vi "MessageBase.setFields.vi"(8 "error in (no error)":errorcluster, 10 "Cluster (dup)":variant, 11 "MessageBase in":refnum<class "MessageBase.lvclass">) -> (0 "error out":errorcluster, 3 "MessageBase out":refnum<class "MessageBase.lvclass">)   [LabVIEW 2022 SP3, in "MessageBase.lvclass"]
uses:
  MessageBase.lvclass
  FieldValue.ctl
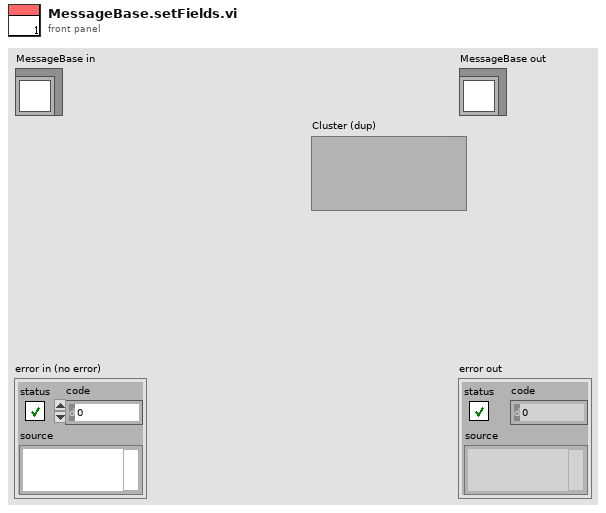
[diagram p1: front panel]
types:
  T1 = typedef "FieldValue.ctl" = variant
  T2 = typedef "FieldSpec.ctl" = cluster{"Name":string, "Offset":i32, "Length":i32, "FieldType":enum16{"Alphanumeric", "Binary", "BinaryLongPrice", "BinaryShortPrice", "BitField", "PrintableAscii", "Value"}, "FieldValue":variant}
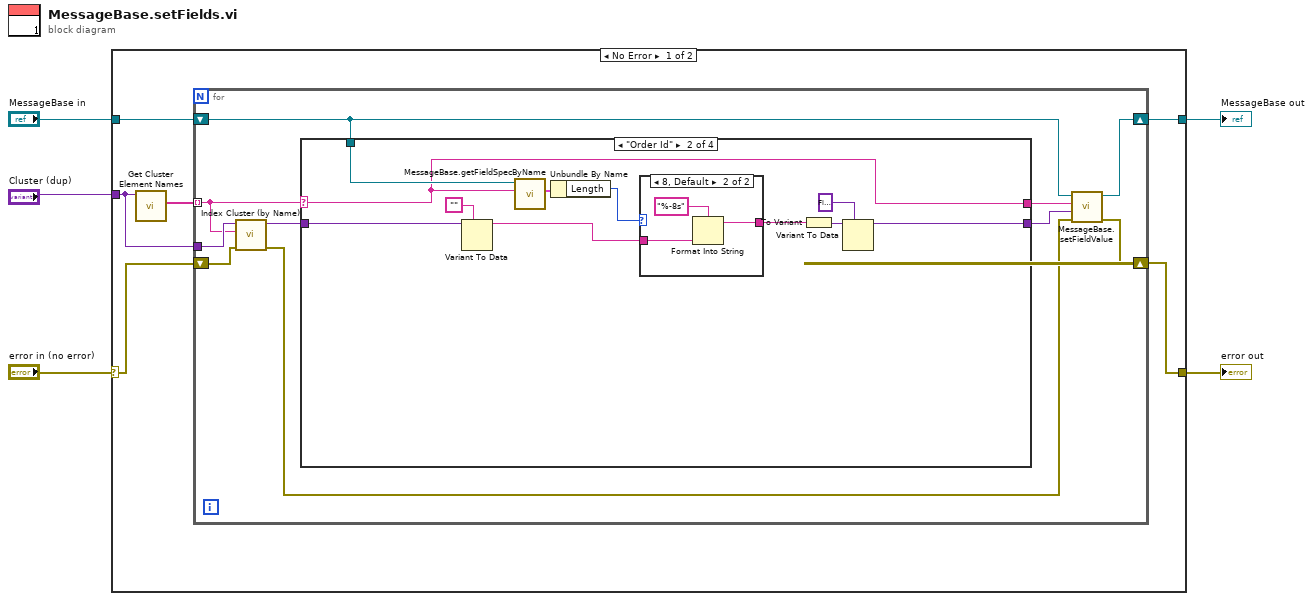
[diagram p0: block diagram]
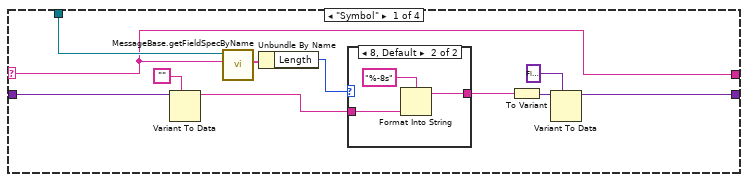
[diagram p2: hidden frame]
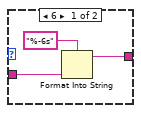
[diagram p3: hidden frame]
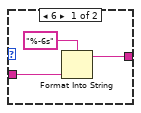
[diagram p4: hidden frame]
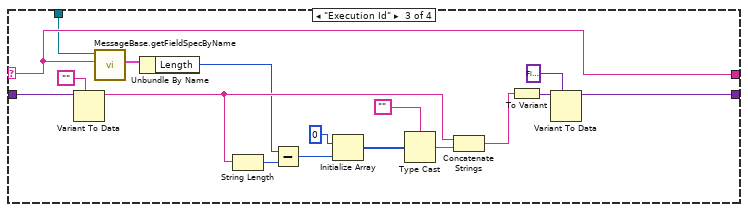
[diagram p5: hidden frame]
diagram:
  n1 = case shown="No Error" "error in (no error)" {
    selector: "error in (no error)" -> [w9 w76]
    tunnel: [w8 w76] -> w4
    tunnel: [w6 w75] -> w2
    tunnel: "MessageBase in" -> [w7 w75]
    tunnel: "Cluster (dup)" -> [w10 _]
    frame No Error {
      n2 = call <vilib>:"Get Cluster Element Names.vi"("Cluster"=w10) -> ("Names"=w11:string[])  [unwired: 8 in, 2 out]
      n3 = for {
        tunnel: w11 -> [w17] mode=indexing
        tunnel: w10 -> [w21]
        shift-right: [w20] -> w6
        shift-left: w7 -> [w12]
        shift-right: [w19] -> w8
        shift-left: w9 -> [w18]
        n4 = call <vilib>:"Index Cluster (by Name).vi"("error in (no error)"=w18, "Element Name"=w17, "Cluster"=w21) -> ("error out"=w13:errorcluster, "Element"=w14:variant)  [unwired: 5 in, 2 out]
        n5 = case shown="\"Order Id\"" w17 {
          selector: w17 -> [w24 w41 w68 w74]
          tunnel: [w24 w41 w68 w74] -> w16
          tunnel: [w30 w47 w70 w73] -> w15
          tunnel: w14 -> [w28 w45 w69 w73]
          tunnel: w12 -> [w25 w42 w56 _]
          frame "Symbol" {
            n6 = Variant To Data(type="", Variant=w28) -> (data=w26:string)  [unwired: 1 in, 1 out]
            n7 = call-dynamic "MessageBase.getFieldSpecByName.vi"("Field.Name"=w24, "MessageBase in"=w25) -> ("FIeldSpec"=w23:T2)  [unwired: 7 in, 2 out]
            n8 = Unbundle By Name(w23) -> ("Length"=w22:i32)
            n9 = case shown="8, Default" w22 {
              tunnel: [w35 w38] -> w29
              tunnel: w26 -> [w33 w36]
              frame 6 {
                n10 = Format Into String(format string="%-6s", w33) -> (resulting string=w35:string)  [unwired: 2 in, 1 out]
              }
              frame 8, Default {
                n11 = Format Into String(format string="%-8s", w36) -> (resulting string=w38:string)  [unwired: 2 in, 1 out]
              }
            }
            n12 = To Variant(anything=w29) -> (Variant=w32:variant)
            n13 = Variant To Data(type=T1 variant ("FieldValue"), Variant=w32) -> (data=w30:T1)  [unwired: 1 in, 1 out]
          }
          frame "Order Id" {
            n14 = Variant To Data(type="", Variant=w45) -> (data=w43:string)  [unwired: 1 in, 1 out]
            n15 = call-dynamic "MessageBase.getFieldSpecByName.vi"("Field.Name"=w41, "MessageBase in"=w42) -> ("FIeldSpec"=w40:T2)  [unwired: 7 in, 2 out]
            n16 = Unbundle By Name(w40) -> ("Length"=w39:i32)
            n17 = case shown="8, Default" w39 {
              tunnel: [w52 w55] -> w46
              tunnel: w43 -> [w50 w53]
              frame 6 {
                n18 = Format Into String(format string="%-6s", w50) -> (resulting string=w52:string)  [unwired: 2 in, 1 out]
              }
              frame 8, Default {
                n19 = Format Into String(format string="%-8s", w53) -> (resulting string=w55:string)  [unwired: 2 in, 1 out]
              }
            }
            n20 = To Variant(anything=w46) -> (Variant=w49:variant)
            n21 = Variant To Data(type=T1 variant ("FieldValue"), Variant=w49) -> (data=w47:T1)  [unwired: 1 in, 1 out]
          }
          frame "Execution Id" {
            n22 = Variant To Data(type="", Variant=w69) -> (data=w59:string)  [unwired: 1 in, 1 out]
            n23 = call-dynamic "MessageBase.getFieldSpecByName.vi"("Field.Name"=w68, "MessageBase in"=w56) -> ("FIeldSpec"=w66:T2)  [unwired: 7 in, 2 out]
            n24 = Unbundle By Name(w66) -> ("Length"=w58:i32)
            n25 = String Length(string=w59) -> (length=w64:i32)
            n26 = Subtract(x=w58, y=w64) -> (x-y=w63:i32)
            n27 = Initialize Array(u8 0, w63) -> (w62:u8[])
            n28 = Type Cast(type="", x=w62) -> (*(type *) &x=w60:string)
            n29 = Concatenate Strings(w59, w60) -> (w57:string)
            n30 = To Variant(anything=w57) -> (Variant=w72:variant)
            n31 = Variant To Data(type=T1 variant ("FieldValue"), Variant=w72) -> (data=w70:T1)  [unwired: 1 in, 1 out]
          }
          frame "Other", Default {
          }
        }
        n32 = call-dynamic "MessageBase.setFieldValue.vi"("error in (no error)"=w13, "Value"=w15, "FIeld.Name"=w16, "MessageBase in"=w12) -> ("error out"=w19:errorcluster, "MessageBase out"=w20:refnum<class "MessageBase.lvclass">)  [unwired: 6 in]
      }
    }
    frame Error {
    }
  }
  "error out" <- w4
  "MessageBase out" <- w2
